vi "Initialize.vi"(7 "Baud Rate (make sure matches instrument)":u32(ring)=115200 items=["4800"=4600, "9600"=9600, "19200"=19200, "38400"=38400, "57600"=57600, "115200"=115200], 8 "error in (no error)":errorcluster, 9 "Reset? (T: Yes)":bool, 10 "ID Query? (T: Yes)":bool=TRUE, 11 "VISA resource name":refnum<visa-resource-name>="QCpulseGen") -> (0 "error out":errorcluster, 3 "VISA resource name out":refnum<visa-resource-name>)   [LabVIEW 2012, in "Quantum Composers 9000 Series.lvlib"]
doc: "This VI passes the addressing information in the instrument decriptor to the Instr Open VI and returns the instrument ID. You can optionally reset the instrument by setting the front panel reset control. You must run this VI before using any of the instrument driver VIs for this instrument."
uses:
  Quantum Composers 9000 Series.lvlib
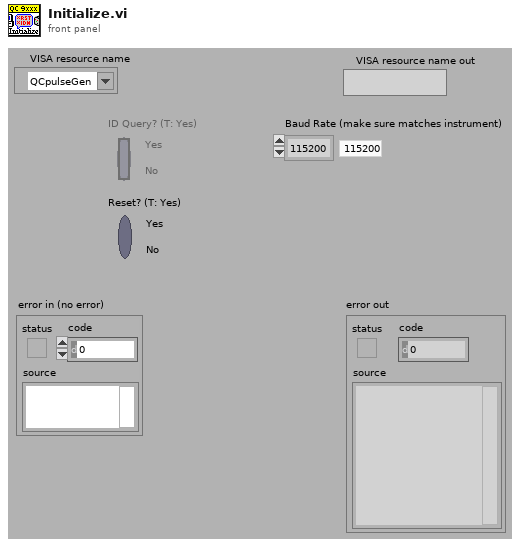
[diagram p1: front panel]
types:
  T1 = enum16{"Read Data", "Write Data", "Dispose of Data", "Clear ALL Data"}
  T2 = typedef "Quantum Composers 9000 Series.lvlib/Unit Info.ctl" = cluster{"ID String":string, "Model":string, "Model #":i32, "# Channels":i32, "Options":string, "Firmware":string, "FPGA Ver":string}
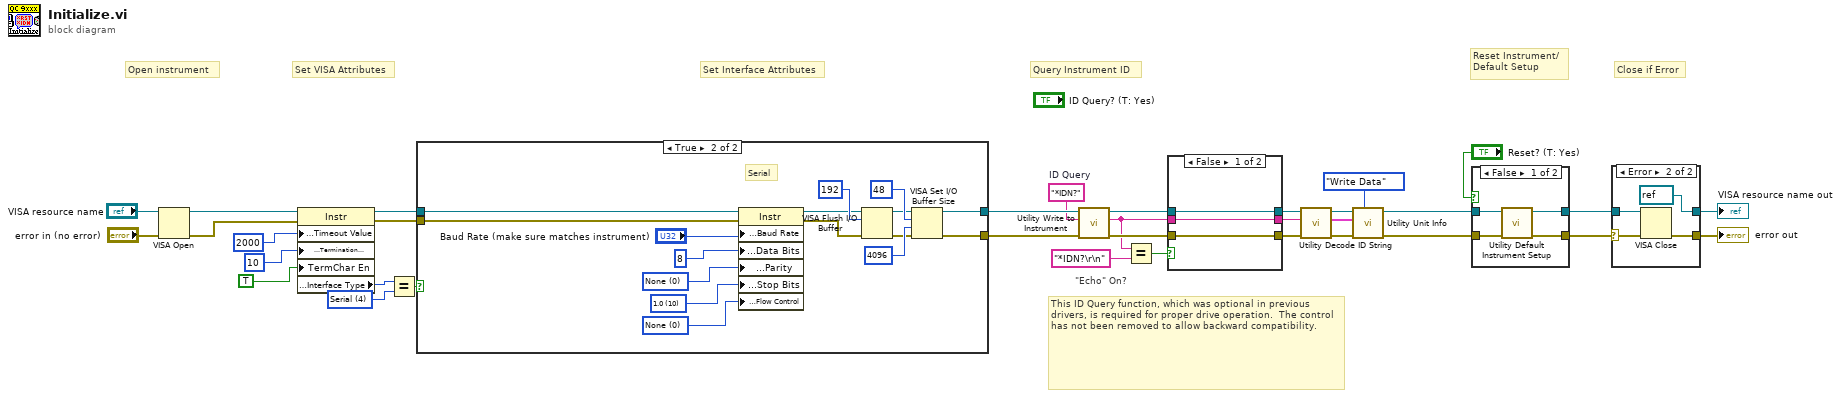
[diagram p0: block diagram]
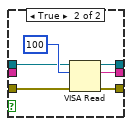
[diagram p2: hidden frame]
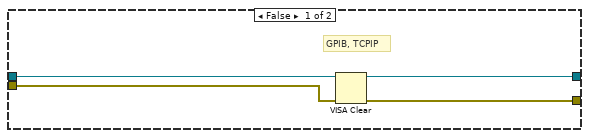
[diagram p3: hidden frame]
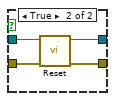
[diagram p5: hidden frame]
diagram:
  w13 = "*IDN?"  # ID Query
  w17 = u16 4 items=["GPIB"=1, "VXI"=2, "GPIB-VXI"=3, "Serial"=4, "PXI"=5, "TCPIP"=6, "USB"=7, "FireWire"=9] ("Interface Information:Interface Type")
  # "This ID Query function, which was optional in previous drivers, is required for proper drive operation.  The control has not been removed to allow backward compatibility."
  # "\"Echo\" On?"
  # "Set Interface Attributes"
  # "Set VISA Attributes"
  # "Close if Error"
  # "Query Instrument ID"
  # "Reset Instrument/\nDefault Setup"
  # "Open instrument"
  n1 = VISA Open(error in (no error)="error in (no error)", VISA resource name="VISA resource name") -> (VISA resource name=w28:refnum<visa-resource-name>, error out=w27:errorcluster)  [unwired: 3 out]
  n2 = property class="Instr"(reference=w28, error in=w27, "General Settings:Timeout Value"=u32 2000, "Message Based Settings:Termination Character"=u8 10, "TermChar En"=TRUE ("Message Based Settings:Termination Character Enable")) -> (reference out=w24:refnum<visa-resource-name>, error out=w25:errorcluster, "Interface Information:Interface Type"=w15:u16)
  n3 = Equal?(x=w15, y=w17) -> (x = y?=w16:bool)
  n4 = case shown="True" w16 {
    tunnel: [w38 w42] -> w22
    tunnel: [w35 w43] -> w21
    tunnel: w24 -> [w37 w53]
    tunnel: w25 -> [w36 w54]
    frame False {
      # "GPIB, TCPIP"
      n5 = VISA Clear(VISA resource name=w37, error in (no error)=w36) -> (VISA resource name out=w38:refnum<visa-resource-name>, error out=w35:errorcluster)
    }
    frame True {
      w49 = u16 0 items=["None"=0, "XON/XOFF"=1, "RTS/CTS"=2, "DTR/DSR"=4] ("Serial Settings:Serial Flow Control")
      w50 = u16 10 items=["1.0"=10, "1.5"=15, "2.0"=20] ("Serial Settings:Serial Stop Bits")
      w51 = u16 0 items=["None", "Odd", "Even", "Mark", "Space"] ("Serial Settings:Serial Parity")
      # "Serial"
      n6 = property class="Instr"(reference=w53, error in=w54, "Serial Settings:Baud Rate"="Baud Rate (make sure matches instrument)", "Serial Settings:Data Bits"=u16 8 ("Serial Settings:Serial Data Bits"), "Serial Settings:Parity"=w51, "Serial Settings:Stop Bits"=w50, "Serial Settings:Flow Control"=w49) -> (reference out=w41:refnum<visa-resource-name>, error out=w40:errorcluster)
      n7 = VISA Flush I/O Buffer(VISA resource name=w41, mask (16)=u16 192, error in (no error)=w40) -> (VISA resource name out=w44:refnum<visa-resource-name>, error out=w45:errorcluster)
      n8 = VISA Set I/O Buffer Size(VISA resource name=w44, mask (16)=u16 48, size (4096)=u32 4096 ("size (0)"), error in (no error)=w45) -> (VISA resource name out=w42:refnum<visa-resource-name>, error out=w43:errorcluster)
    }
  }
  n9 = call "Utility Write to Instrument.vi"("error in (no error)"=w21, "Write Buffer"=w13, "VISA resource name"=w22) -> ("error out"=w11:errorcluster, "Read Buffer"=w9:string, "VISA resource name out"=w12:refnum<visa-resource-name>)  [unwired: 6 out]
  n10 = Equal?(x=w9, y="*IDN?\r\n") -> (x = y?=w8:bool)
  n11 = case shown="False" w8 {
    tunnel: w12 -> [w57 w59]
    tunnel: w11 -> [w56 w61]
    tunnel: [w57 w63] -> w5
    tunnel: [w56 w60] -> w6
    tunnel: [w55 w58] -> w1
    tunnel: w9 -> [w55 _]
    frame False {
    }
    frame True {
      n12 = VISA Read(VISA resource name=w59, byte count=u32 100 ("byte count (0)"), error in (no error)=w61) -> (VISA resource name out=w63:refnum<visa-resource-name>, read buffer=w58:string, error out=w60:errorcluster)  [unwired: 1 out]
    }
  }
  n13 = call "Utility Decode ID String.vi"("error in (no error)"=w6, "*IDN? Response"=w1, "VISA resource name in"=w5) -> ("error out"=w7:errorcluster, "Unit Info"=w3:T2, "VISA resource name out"=w4:refnum<visa-resource-name>)  [unwired: 6 out]
  n14 = call "Utility Unit Info.vi"("Action"=T1."Write Data", "Error In (no error)"=w7, "Unit Info In"=w3, "VISA resource name in"=w4) -> ("Error Out"=w33:errorcluster, "VISA resource name out"=w34:refnum<visa-resource-name>)  [unwired: 6 out]
  n15 = case shown="False" "Reset? (T: Yes)" {
    tunnel: w33 -> [w66 w68]
    tunnel: [w65 w71] -> w20
    tunnel: w34 -> [w67 w69]
    tunnel: [w64 w70] -> w31
    frame False {
      n16 = call "Utility Default Instrument Setup.vi"("error in (no error)"=w66, "VISA resource name"=w67) -> ("error out"=w65:errorcluster, "VISA resource name out"=w64:refnum<visa-resource-name>)  [unwired: 8 out]
    }
    frame True {
      n17 = call "Reset.vi"("error in (no error)"=w68, "VISA resource name"=w69) -> ("error out"=w71:errorcluster, "VISA resource name out"=w70:refnum<visa-resource-name>)  [unwired: 8 out]
    }
  }
  n18 = case shown="Error" w20 {
    selector: w20 -> [w72 w76]
    tunnel: w31 -> [w73 w75]
    tunnel: [w73 refnum<visa-resource-name> refnum ("dup VISA resource")] -> w30
    tunnel: [w72 w77] -> w29
    frame No Error {
    }
    frame Error {
      n19 = VISA Close(VISA resource name=w75, error in (no error)=w76) -> (error out=w77:errorcluster)
    }
  }
  "error out" <- w29
  "VISA resource name out" <- w30
